vi "test_read-nmea-data2.vi"() -> ()   [LabVIEW 2019] (continued)
\n15:13:53.49\tF9P\t$GLGSV,2,1,08,69,11,031,33,70,70,038,25,71,53,206,32,72,05,210,17,1*72\n\t\n15:13:53.51\tF9P\t$GLGSV,2,2,08,77,01,325,,84,19,123,24,85,70,070,34,86,37,330,,1*77\n\t\n15:13:53.53\tF9P\t$GLGSV,2,1,08,69,11,031,31,70,70,038,,71,53,206,25,72,05,210,,3*75\n\t\n15:13:53.55\tF9P\t$GLGSV,2,2,08,77,01,325,,84,19,123,30,85,70,070,24,86,37,330,,3*71\n\t\n15:13:53.57\tF9P\t$GAGSV,2,1,08,02,08,296,12,04,67,115,32,09,32,193,20,11,72,359,26,7*72\n\t\n15:13:53.59\tF9P\t$GAGSV,2,2,08,12,40,103,28,19,26,045,19,25,09,249,10,36,26,308,12,7*78\n\t\n15:13:53.61\tF9P\t$GAGSV,2,1,08,02,08,296,,04,67,115,,09,32,193,,11,72,359,,2*73\n\t\n15:13:53.63\tF9P\t$GAGSV,2,2,08,12,40,103,,19,26,045,,25,09,249,,36,26,308,,2*7D\n\t\n15:13:53.65\tF9P\t$GBGSV,1,1,04,11,49,132,36,14,87,114,26,28,,,27,33,61,220,30,1*4B\n\t\n15:13:53.67\tF9P\t$GBGSV,1,1,03,11,49,132,33,14,87,114,,33,61,220,,3*43\n\t\n15:13:53.69\tF9P\t$GNGLL,3723.57673,N,12656.98677,E,061355.00,A,A*77\n\t\n15:13:53.71\tF9P\t\t\n15:13:53.73\tF9P\t\t\n15:13:53.75\tF9P\t\t\n15:13:53.77\tF9P\t\t\n15:13:53.79\tF9P\t\t\n15:13:53.81\tF9P\t\t\n15:13:53.83\tF9P\t\t\n15:13:53.85\tF9P\t\t\n15:13:53.87\tF9P\t\t\n15:13:53.89\tF9P\t\t\n15:13:53.91\tF9P\t\t\n15:13:53.93\tF9P\t\t\n15:13:53.95\tF9P\t\t\n15:13:53.97\tF9P\t\t\n15:13:53.99\tF9P\t\t\n15:13:54.01\tF9P\t\t\n15:13:54.03\tF9P\t\t\n15:13:54.05\tF9P\t\t\n15:13:54.07\tF9P\t\t\n15:13:54.09\tF9P\t\t\n15:13:54.11\tF9P\t\t\n15:13:54.13\tF9P\t\t\n15:13:54.15\tF9P\t\t\n15:13:54.17\tF9P\t\t\n15:13:54.19\tF9P\t\t\n15:13:54.21\tF9P\t\t\n15:13:54.23\tF9P\t$GNRMC,061356.00,A,3723.57755,N,12656.98651,E,2.289,328.38,250720,,,A,V*09\n\t\n15:13:54.25\tF9P\t$GNVTG,328.38,T,,M,2.289,N,4.239,K,A*2C\n\t\n15:13:54.27\tF9P\t$GNGGA,061356.00,3723.57755,N,12656.98651,E,1,12,0.74,48.4,M,18.5,M,,*74\n\t\n15:13:54.29\tF9P\t$GNGSA,A,3,12,06,19,05,17,09,04,02,,,,,1.37,0.74,1.15,1*03\n\t\n15:13:54.31\tF9P\t$GNGSA,A,3,85,70,71,84,,,,,,,,,1.37,0.74,1.15,2*01\n\t\n15:13:54.33\tF9P\t$GNGSA,A,3,36,19,11,04,09,12,,,,,,,1.37,0.74,1.15,3*03\n\t\n15:13:54.35\tF9P\t$GNGSA,A,3,14,11,33,,,,,,,,,,1.37,0.74,1.15,4*02\n\t\n15:13:54.37\tF9P\t$GPGSV,3,1,09,02,55,320,27,04,17,043,23,05,38,248,23,06,64,050,29,1*66\n\t\n15:13:54.39\tF9P\t$GPGSV,3,2,09,09,44,073,29,12,23,276,25,17,32,154,33,19,51,157,35,1*62\n\t\n15:13:54.41\tF9P\t$GPGSV,3,3,09,25,12,306,23,1*5D\n\t\n15:13:54.43\tF9P\t$GPGSV,3,1,09,02,55,320,,04,17,043,,05,38,248,18,06,64,050,23,6*67\n\t\n15:13:54.45\tF9P\t$GPGSV,3,2,09,09,44,073,30,12,23,276,,17,32,154,19,19,51,157,,6*64\n\t\n15:13:54.47\tF9P\t$GPGSV,3,3,09,25,12,306,,6*5B\n\t\n15:13:54.49\tF9P\t$GLGSV,2,1,08,69,11,031,34,70,70,038,25,71,53,206,32,72,05,210,17,1*75\n\t\n15:13:54.51\tF9P\t$GLGSV,2,2,08,77,01,325,,84,19,123,26,85,70,070,39,86,37,330,,1*78\n\t\n15:13:54.53\tF9P\t$GLGSV,2,1,08,69,11,031,26,70,70,038,,71,53,206,23,72,05,210,,3*75\n\t\n15:13:54.55\tF9P\t$GLGSV,2,2,08,77,01,325,,84,19,123,33,85,70,070,23,86,37,330,,3*75\n\t\n15:13:54.57\tF9P\t$GAGSV,2,1,08,02,08,296,10,04,67,115,40,09,32,193,21,11,72,359,26,7*74\n\t\n15:13:54.59\tF9P\t$GAGSV,2,2,08,12,40,103,33,19,26,045,20,25,09,249,13,36,26,308,13,7*7A\n\t\n15:13:54.61\tF9P\t$GAGSV,2,1,08,02,08,296,,04,67,115,,09,32,193,,11,72,359,,2*73\n\t\n15:13:54.63\tF9P\t$GAGSV,2,2,08,12,40,103,,19,26,045,,25,09,249,,36,26,308,,2*7D\n\t\n15:13:54.65\tF9P\t$GBGSV,1,1,04,11,49,132,30,14,87,114,32,28,,,25,33,61,220,29,1*42\n\t\n15:13:54.67\tF9P\t$GBGSV,1,1,03,11,49,132,32,14,87,114,29,33,61,220,,3*49\n\t\n15:13:54.69\tF9P\t$GNGLL,3723.57755,N,12656.98651,E,061356.00,A,A*75\n\t\n15:13:54.71\tF9P\t\t\n15:13:54.73\tF9P\t\t\n15:13:54.75\tF9P\t\t\n15:13:54.77\tF9P\t\t\n15:13:54.79\tF9P\t\t\n15:13:54.81\tF9P\t\t\n15:13:54.83\tF9P\t\t\n15:13:54.85\tF9P\t\t\n15:13:54.87\tF9P\t\t\n15:13:54.89\tF9P\t\t\n15:13:54.91\tF9P\t\t\n15:13:54.93\tF9P\t\t\n15:13:54.95\tF9P\t\t\n15:13:54.97\tF9P\t\t\n15:13:54.99\tF9P\t\t\n15:13:55.01\tF9P\t\t\n15:13:55.03\tF9P\t\t\n15:13:55.05\tF9P\t\t\n15:13:55.07\tF9P\t\t\n15:13:55.09\tF9P\t\t\n15:13:55.11\tF9P\t\t\n15:13:55.13\tF9P\t\t\n15:13:55.15\tF9P\t\t\n15:13:55.17\tF9P\t\t\n15:13:55.19\tF9P\t\t\n15:13:55.21\tF9P\t\t\n15:13:55.23\tF9P\t$GNRMC,061357.00,A,3723.57810,N,12656.98637,E,2.065,333.34,250720,,,A,V*00\n\t\n15:13:55.25\tF9P\t$GNVTG,333.34,T,,M,2.065,N,3.825,K,A*2A\n\t\n15:13:55.27\tF9P\t$GNGGA,061357.00,3723.57810,N,12656.98637,E,1,12,0.70,48.3,M,18.5,M,,*78\n\t\n15:13:55.29\tF9P\t$GNGSA,A,3,12,06,19,05,17,09,04,02,,,,,1.27,0.70,1.06,1*04\n\t\n15:13:55.31\tF9P\t$GNGSA,A,3,85,70,71,84,,,,,,,,,1.27,0.70,1.06,2*06\n\t\n15:13:55.33\tF9P\t$GNGSA,A,3,36,19,11,04,09,12,,,,,,,1.27,0.70,1.06,3*04\n\t\n15:13:55.35\tF9P\t$GNGSA,A,3,14,11,33,,,,,,,,,,1.27,0.70,1.06,4*05\n\t\n15:13:55.37\tF9P\t$GPGSV,3,1,09,02,55,320,25,04,17,043,24,05,38,248,34,06,64,050,29,1*65\n\t\n15:13:55.39\tF9P\t$GPGSV,3,2,09,09,44,073,29,12,23,276,25,17,32,154,40,19,51,157,28,1*6A\n\t\n15:13:55.41\tF9P\t$GPGSV,3,3,09,25,12,306,19,1*54\n\t\n15:13:55.43\tF9P\t$GPGSV,3,1,09,02,55,320,,04,17,043,20,05,38,248,20,06,64,050,22,6*6F\n\t\n15:13:55.45\tF9P\t$GPGSV,3,2,09,09,44,073,23,12,23,276,,17,32,154,23,19,51,157,,6*6F\n\t\n15:13:55.47\tF9P\t$GPGSV,3,3,09,25,12,306,,6*5B\n\t\n15:13:55.49\tF9P\t$GLGSV,2,1,08,69,11,031,26,70,70,038,24,71,53,206,27,72,05,210,17,1*73\n\t\n15:13:55.51\tF9P\t$GLGSV,2,2,08,77,01,325,,84,19,123,31,85,70,070,32,86,37,330,,1*75\n\t\n15:13:55.53\tF9P\t$GLGSV,2,1,08,69,11,031,25,70,70,038,,71,53,206,22,72,05,210,,3*77\n\t\n15:13:55.55\tF9P\t$GLGSV,2,2,08,77,01,325,,84,19,123,32,85,70,070,22,86,37,330,,3*75\n\t\n15:13:55.57\tF9P\t$GAGSV,2,1,08,02,08,296,10,04,67,115,27,09,33,193,21,11,72,359,26,7*74\n\t\n15:13:55.59\tF9P\t$GAGSV,2,2,08,12,40,103,29,19,26,045,19,25,09,249,15,36,26,308,11,7*7F\n\t\n15:13:55.61\tF9P\t$GAGSV,2,1,08,02,08,296,,04,67,115,,09,33,193,,11,72,359,,2*72\n\t\n15:13:55.63\tF9P\t$GAGSV,2,2,08,12,40,103,,19,26,045,,25,09,249,,36,26,308,,2*7D\n\t\n15:13:55.65\tF9P\t$GBGSV,1,1,04,11,49,132,27,14,87,114,31,28,,,27,33,61,220,36,1*4B\n\t\n15:13:55.67\tF9P\t$GBGSV,1,1,04,08,,,36,11,49,132,32,14,87,114,34,33,61,220,,3*4F\n\t\n15:13:55.69\tF9P\t$GNGLL,3723.57810,N,12656.98637,E,061357.00,A,A*7A\n\t\n15:13:55.71\tF9P\t\t\n15:13:55.73\tF9P\t\t\n15:13:55.75\tF9P\t\t\n15:13:55.77\tF9P\t\t\n15:13:55.79\tF9P\t\t\n15:13:55.81\tF9P\t\t\n15:13:55.83\tF9P\t\t\n15:13:55.85\tF9P\t\t\n15:13:55.87\tF9P\t\t\n15:13:55.89\tF9P\t\t\n15:13:55.91\tF9P\t\t\n15:13:55.93\tF9P\t\t\n15:13:55.95\tF9P\t\t\n15:13:55.97\tF9P\t\t\n15:13:55.99\tF9P\t\t\n15:13:56.01\tF9P\t\t\n15:13:56.03\tF9P\t\t\n15:13:56.05\tF9P\t\t\n15:13:56.07\tF9P\t\t\n15:13:56.09\tF9P\t\t\n15:13:56.11\tF9P\t\t\n15:13:56.13\tF9P\t\t\n15:13:56.15\tF9P\t\t\n15:13:56.17\tF9P\t\t\n15:13:56.19\tF9P\t\t\n15:13:56.21\tF9P\t\t\n15:13:56.23\tF9P\t$GNRMC,061358.00,A,3723.57882,N,12656.98586,E,2.274,334.11,250720,,,A,V*0F\n\t\n15:13:56.25\tF9P\t$GNVTG,334.11,T,,M,2.274,N,4.211,K,A*22\n\t\n15:13:56.27\tF9P\t$GNGGA,061358.00,3723.57882,N,12656.98586,E,1,12,0.74,47.8,M,18.5,M,,*75\n\t\n15:13:56.29\tF9P\t$GNGSA,A,3,12,06,19,05,17,09,04,02,,,,,1.37,0.74,1.15,1*03\n\t\n15:13:56.31\tF9P\t$GNGSA,A,3,85,70,71,84,,,,,,,,,1.37,0.74,1.15,2*01\n\t\n15:13:56.33\tF9P\t$GNGSA,A,3,36,19,11,04,09,12,,,,,,,1.37,0.74,1.15,3*03\n\t\n15:13:56.35\tF9P\t$GNGSA,A,3,14,11,33,,,,,,,,,,1.37,0.74,1.15,4*02\n\t\n15:13:56.37\tF9P\t$GPGSV,3,1,09,02,55,320,25,04,17,043,24,05,38,248,42,06,64,050,33,1*6F\n\t\n15:13:56.39\tF9P\t$GPGSV,3,2,09,09,44,073,33,12,23,276,30,17,32,154,36,19,51,157,33,1*6E\n\t\n15:13:56.41\tF9P\t$GPGSV,3,3,09,25,12,306,18,1*55\n\t\n15:13:56.43\tF9P\t$GPGSV,3,1,09,02,55,320,,04,17,043,18,05,38,248,22,06,64,050,24,6*60\n\t\n15:13:56.45\tF9P\t$GPGSV,3,2,09,09,44,073,23,12,23,276,,17,32,154,22,19,51,157,19,6*66\n\t\n15:13:56.47\tF9P\t$GPGSV,3,3,09,25,12,306,,6*5B\n\t\n15:13:56.49\tF9P\t$GLGSV,2,1,08,69,11,031,30,70,70,038,22,71,53,206,30,72,05,210,17,1*74\n\t\n15:13:56.51\tF9P\t$GLGSV,2,2,08,77,01,325,,84,19,123,28,85,70,070,27,86,37,330,,1*79\n\t\n15:13:56.53\tF9P\t$GLGSV,2,1,08,69,11,031,23,70,70,038,,71,53,206,27,72,05,210,,3*74\n\t\n15:13:56.55\tF9P\t$GLGSV,2,2,08,77,01,325,,84,19,123,35,85,70,070,21,86,37,330,,3*71\n\t\n15:13:56.57\tF9P\t$GAGSV,2,1,08,02,08,296,08,04,67,115,30,09,33,193,22,11,72,001,26,7*76\n\t\n15:13:56.59\tF9P\t$GAGSV,2,2,08,12,40,103,23,19,26,045,21,25,09,249,15,36,26,308,13,7*7C\n\t\n15:13:56.61\tF9P\t$GAGSV,2,1,08,02,08,296,,04,67,115,,09,33,193,,11,72,001,,2*7C\n\t\n15:13:56.63\tF9P\t$GAGSV,2,2,08,12,40,103,,19,26,045,,25,09,249,,36,26,308,,2*7D\n\t\n15:13:56.65\tF9P\t$GBGSV,1,1,04,11,49,132,32,14,87,114,32,28,,,31,33,61,220,36,1*4B\n\t\n15:13:56.67\tF9P\t$GBGSV,1,1,04,08,,,33,11,49,132,30,14,87,114,34,33,61,220,,3*48\n\t\n15:13:56.69\tF9P\t$GNGLL,3723.57882,N,12656.98586,E,061358.00,A,A*77\n\t\n15:13:56.71\tF9P\t\t\n15:13:56.73\tF9P\t\t\n15:13:56.75\tF9P\t\t\n15:13:56.77\tF9P\t\t\n15:13:56.79\tF9P\t\t\n15:13:56.81\tF9P\t\t\n15:13:56.83\tF9P\t\t\n15:13:56.85\tF9P\t\t\n15:13:56.87\tF9P\t\t\n15:13:56.89\tF9P\t\t\n15:13:56.91\tF9P\t\t\n15:13:56.93\tF9P\t\t\n15:13:56.95\tF9P\t\t\n15:13:56.97\tF9P\t\t\n15:13:56.99\tF9P\t\t\n15:13:57.01\tF9P\t\t\n15:13:57.03\tF9P\t\t\n15:13:57.05\tF9P\t\t\n15:13:57.07\tF9P\t\t\n15:13:57.09\tF9P\t\t\n15:13:57.11\tF9P\t\t\n15:13:57.13\tF9P\t\t\n15:13:57.15\tF9P\t\t\n15:13:57.17\tF9P\t\t\n15:13:57.19\tF9P\t\t\n15:13:57.21\tF9P\t\t\n15:13:57.23\tF9P\t$GNRMC,061359.00,A,3723.57946,N,12656.98547,E,2.498,332.08,250720,,,A,V*00\n\t\n15:13:57.25\tF9P\t$GNVTG,332.08,T,,M,2.498,N,4.627,K,A*29\n\t\n15:13:57.27\tF9P\t$GNGGA,061359.00,3723.57946,N,12656.98547,E,1,12,0.74,47.9,M,18.5,M,,*71\n\t\n15:13:57.29\tF9P\t$GNGSA,A,3,12,06,19,05,17,09,04,02,,,,,1.37,0.74,1.15,1*03\n\t\n15:13:57.31\tF9P\t$GNGSA,A,3,85,70,71,84,,,,,,,,,1.37,0.74,1.15,2*01\n\t\n15:13:57.33\tF9P\t$GNGSA,A,3,36,19,11,04,09,12,,,,,,,1.37,0.74,1.15,3*03\n\t\n15:13:57.35\tF9P\t$GNGSA,A,3,14,11,33,,,,,,,,,,1.37,0.74,1.15,4*02\n\t\n15:13:57.37\tF9P\t$GPGSV,3,1,09,02,55,320,28,04,17,043,25,05,38,248,28,06,64,050,40,1*6B\n\t\n15:13:57.39\tF9P\t$GPGSV,3,2,09,09,44,073,29,12,23,276,22,17,32,154,40,19,51,157,22,1*67\n\t\n15:13:57.41\tF9P\t$GPGSV,3,3,09,25,12,306,18,1*55\n\t\n15:13:57.43\tF9P\t$GPGSV,3,1,09,02,55,320,,04,17,043,15,05,38,248,20,06,64,050,22,6*69\n\t\n15:13:57.45\tF9P\t$GPGSV,3,2,09,09,44,073,21,12,23,276,18,17,32,154,21,19,51,157,16,6*61\n\t\n15:13:57.47\tF9P\t$GPGSV,3,3,09,25,12,306,,6*5B\n\t\n15:13:57.49\tF9P\t$GLGSV,2,1,08,69,11,031,28,70,70,038,22,71,53,206,30,72,05,210,18,1*72\n\t\n15:13:57.51\tF9P\t$GLGSV,2,2,08,77,01,325,,84,19,123,29,85,70,070,28,86,37,330,,1*77\n\t\n15:13:57.53\tF9P\t$GLGSV,2,1,08,69,11,031,22,70,70,038,,71,53,206,25,72,05,210,,3*77\n\t\n15:13:57.55\tF9P\t$GLGSV,2,2,08,77,01,325,,84,19,123,25,85,70,070,21,86,37,330,,3*70\n\t\n15:13:57.57\tF9P\t$GAGSV,2,1,08,02,08,296,09,04,67,115,23,09,33,193,22,11,72,001,26,7*75\n\t\n15:13:57.59\tF9P\t$GAGSV,2,2,08,12,39,103,25,19,26,045,21,25,09,249,16,36,26,308,12,7*76\n\t\n15:13:57.61\tF9P\t$GAGSV,2,1,08,02,08,296,,04,67,115,,09,33,193,,11,72,001,,2*7C\n\t\n15:13:57.63\tF9P\t$GAGSV,2,2,08,12,39,103,,19,26,045,,25,09,249,,36,26,308,,2*73\n\t\n15:13:57.65\tF9P\t$GBGSV,1,1,04,11,49,132,35,14,87,114,28,28,,,25,33,61,220,32,1*46\n\t\n15:13:57.67\tF9P\t$GBGSV,1,1,04,08,,,30,11,49,132,26,14,87,114,31,33,61,220,,3*49\n\t\n15:13:57.69\tF9P\t$GNGLL,3723.57946,N,12656.98547,E,061359.00,A,A*72\n\t\n15:13:57.71\tF9P\t\t\n15:13:57.73\tF9P\t\t\n15:13:57.75\tF9P\t\t\n15:13:57.77\tF9P\t\t\n15:13:57.79\tF9P\t\t\n15:13:57.81\tF9P\t\t\n15:13:57.83\tF9P\t\t\n15:13:57.85\tF9P\t\t\n15:13:57.87\tF9P\t\t\n15:13:57.89\tF9P\t\t\n15:13:57.91\tF9P\t\t\n15:13:57.93\tF9P\t\t\n15:13:57.95\tF9P\t\t\n15:13:57.97\tF9P\t\t\n15:13:57.99\tF9P\t\t\n15:13:58.01\tF9P\t\t\n15:13:58.03\tF9P\t\t\n15:13:58.05\tF9P\t\t\n15:13:58.07\tF9P\t\t\n15:13:58.09\tF9P\t\t\n15:13:58.11\tF9P\t\t\n15:13:58.13\tF9P\t\t\n15:13:58.15\tF9P\t\t\n15:13:58.17\tF9P\t\t\n15:13:58.19\tF9P\t\t\n15:13:58.21\tF9P\t\t\n15:13:58.23\tF9P\t$GNRMC,061400.00,A,3723.58004,N,12656.98518,E,1.633,332.76,250720,,,A,V*08\n\t\n15:13:58.25\tF9P\t$GNVTG,332.76,T,,M,1.633,N,3.024,K,A*22\n\t\n15:13:58.27\tF9P\t$GNGGA,061400.00,3723.58004,N,12656.98518,E,1,12,0.71,47.9,M,18.5,M,,*75\n\t\n15:13:58.29\tF9P\t$GNGSA,A,3,12,06,19,05,17,09,04,02,,,,,1.33,0.71,1.12,1*05\n\t\n15:13:58.31\tF9P\t$GNGSA,A,3,85,70,71,84,,,,,,,,,1.33,0.71,1.12,2*07\n\t\n15:13:58.33\tF9P\t$GNGSA,A,3,36,19,11,04,09,12,,,,,,,1.33,0.71,1.12,3*05\n\t\n15:13:58.35\tF9P\t$GNGSA,A,3,14,11,33,,,,,,,,,,1.33,0.71,1.12,4*04\n\t\n15:13:58.37\tF9P\t$GPGSV,3,1,09,02,55,320,28,04,17,043,25,05,38,248,41,06,64,050,29,1*6B\n\t\n15:13:58.39\tF9P\t$GPGSV,3,2,09,09,44,073,32,12,23,276,21,17,32,154,30,19,51,157,28,1*63\n\t\n15:13:58.41\tF9P\t$GPGSV,3,3,09,25,12,306,19,1*54\n\t\n15:13:58.43\tF9P\t$GPGSV,3,1,09,02,55,320,,04,17,043,16,05,38,248,29,06,64,050,30,6*60\n\t\n15:13:58.45\tF9P\t$GPGSV,3,2,09,09,44,073,20,12,23,276,15,17,32,154,21,19,51,157,09,6*63\n\t\n15:13:58.47\tF9P\t$GPGSV,3,3,09,25,12,306,,6*5B\n\t\n15:13:58.49\tF9P\t$GLGSV,2,1,08,69,11,031,22,70,70,038,22,71,53,206,23,72,05,210,17,1*75\n\t\n15:13:58.51\tF9P\t$GLGSV,2,2,08,77,01,325,,84,19,123,27,85,70,070,32,86,37,330,,1*72\n\t\n15:13:58.53\tF9P\t$GLGSV,2,1,08,69,11,031,25,70,70,038,,71,53,206,23,72,05,210,,3*76\n\t\n15:13:58.55\tF9P\t$GLGSV,2,2,08,77,01,325,,84,19,123,26,85,70,070,21,86,37,330,,3*73\n\t\n15:13:58.57\tF9P\t$GAGSV,2,1,08,02,08,296,10,04,67,115,25,09,33,193,30,11,72,001,26,7*78\n\t\n15:13:58.59\tF9P\t$GAGSV,2,2,08,12,39,103,24,19,26,045,21,25,09,249,14,36,26,308,14,7*73\n\t\n15:13:58.61\tF9P\t$GAGSV,2,1,08,02,08,296,,04,67,115,,09,33,193,,11,72,001,31,2*7E\n\t\n15:13:58.63\tF9P\t$GAGSV,2,2,08,12,39,103,,19,26,045,,25,09,249,,36,26,308,,2*73\n\t\n15:13:58.65\tF9P\t$GBGSV,1,1,04,11,49,132,28,14,87,114,26,28,,,25,33,61,220,37,1*41\n\t\n15:13:58.67\tF9P\t$GBGSV,1,1,04,08,,,29,11,49,132,,14,87,114,30,33,61,220,,3*44\n\t\n15:13:58.70\tF9P\t$GNGLL,3723.58004,N,12656.98518,E,061400.00,A,A*73\n\t\n15:13:58.72\tF9P\t\t\n15:13:58.74\tF9P\t\t\n15:13:58.76\tF9P\t\t\n15:13:58.78\tF9P\t\t\n15:13:58.80\tF9P\t\t\n15:13:58.82\tF9P\t\t\n15:13:58.84\tF9P\t\t\n15:13:58.86\tF9P\t\t\n15:13:58.88\tF9P\t\t\n15:13:58.90\tF9P\t\t\n15:13:58.92\tF9P\t\t\n15:13:58.94\tF9P\t\t\n15:13:58.96\tF9P\t\t\n15:13:58.98\tF9P\t\t\n15:13:59.00\tF9P\t\t\n15:13:59.02\tF9P\t\t\n15:13:59.04\tF9P\t\t\n15:13:59.06\tF9P\t\t\n15:13:59.08\tF9P\t\t\n15:13:59.10\tF9P\t\t\n15:13:59.12\tF9P\t\t\n15:13:59.14\tF9P\t\t\n15:13:59.16\tF9P\t\t\n15:13:59.18\tF9P\t\t\n15:13:59.20\tF9P\t\t\n15:13:59.22\tF9P\t\t\n15:13:59.24\tF9P\t$GNRMC,061401.00,A,3723.58046,N,12656.98492,E,0.886,335.81,250720,,,A,V*02\n\t\n15:13:59.26\tF9P\t$GNVTG,335.81,T,,M,0.886,N,1.641,K,A*2B\n\t\n15:13:59.28\tF9P\t$GNGGA,061401.00,3723.58046,N,12656.98492,E,1,12,0.71,47.5,M,18.5,M,,*7D\n\t\n15:13:59.30\tF9P\t$GNGSA,A,3,12,06,19,05,17,09,04,02,,,,,1.27,0.71,1.05,1*06\n\t\n15:13:59.32\tF9P\t$GNGSA,A,3,85,70,71,84,,,,,,,,,1.27,0.71,1.05,2*04\n\t\n15:13:59.34\tF9P\t$GNGSA,A,3,36,19,11,04,09,12,,,,,,,1.27,0.71,1.05,3*06\n\t\n15:13:59.36\tF9P\t$GNGSA,A,3,14,11,33,,,,,,,,,,1.27,0.71,1.05,4*07\n\t\n15:13:59.38\tF9P\t$GPGSV,3,1,09,02,55,320,32,04,17,043,26,05,38,248,42,06,64,050,28,1*61\n\t\n15:13:59.40\tF9P\t$GPGSV,3,2,09,09,44,073,33,12,23,276,22,17,32,154,30,19,51,157,27,1*6E\n\t\n15:13:59.42\tF9P\t$GPGSV,3,3,09,25,12,306,18,1*55\n\t\n15:13:59.44\tF9P\t$GPGSV,3,1,09,02,55,320,,04,17,043,19,05,38,248,20,06,64,050,22,6*65\n\t\n15:13:59.46\tF9P\t$GPGSV,3,2,09,09,44,073,23,12,23,276,12,17,32,154,21,19,51,157,08,6*66\n\t\n15:13:59.48\tF9P\t$GPGSV,3,3,09,25,12,306,,6*5B\n\t\n15:13:59.50\tF9P\t$GLGSV,2,1,08,69,11,031,24,70,70,038,24,71,53,206,31,72,05,210,15,1*74\n\t\n15:13:59.52\tF9P\t$GLGSV,2,2,08,77,01,325,,84,19,123,10,85,70,070,33,86,37,330,,1*77\n\t\n15:13:59.54\tF9P\t$GLGSV,2,1,08,69,11,031,23,70,70,038,,71,53,206,26,72,05,210,,3*75\n\t\n15:13:59.56\tF9P\t$GLGSV,2,2,08,77,01,325,,84,19,123,25,85,70,070,20,86,37,330,,3*71\n\t\n15:13:59.58\tF9P\t$GAGSV,2,1,08,02,08,296,11,04,67,115,31,09,33,193,23,11,72,001,34,7*7D\n\t\n15:13:59.60\tF9P\t$GAGSV,2,2,08,12,39,103,24,19,26,045,23,25,09,249,11,36,26,308,17,7*77\n\t\n15:13:59.62\tF9P\t$GAGSV,2,1,08,02,08,296,,04,67,115,,09,33,193,,11,72,001,,2*7C\n\t\n15:13:59.64\tF9P\t$GAGSV,2,2,08,12,39,103,,19,26,045,,25,09,249,,36,26,308,,2*73\n\t\n15:13:59.66\tF9P\t$GBGSV,1,1,04,11,49,132,28,14,87,114,32,28,,,31,33,61,220,26,1*41\n\t\n15:13:59.68\tF9P\t$GBGSV,1,1,04,08,,,33,11,49,132,26,14,87,114,29,33,61,220,,3*43\n\t\n15:13:59.70\tF9P\t$GNGLL,3723.58046,N,12656.98492,E,061401.00,A,A*77\n\t\n15:13:59.72\tF9P\t\t\n15:13:59.74\tF9P\t\t\n15:13:59.76\tF9P\t\t\n15:13:59.78\tF9P\t\t\n15:13:59.80\tF9P\t\t\n15:13:59.82\tF9P\t\t\n15:13:59.84\tF9P\t\t\n15:13:59.86\tF9P\t\t\n15:13:59.88\tF9P\t\t\n15:13:59.90\tF9P\t\t\n15:13:59.92\tF9P\t\t\n15:13:59.94\tF9P\t\t\n15:13:59.96\tF9P\t\t\n15:13:59.98\tF9P\t\t\n15:14:00.00\tF9P\t\t\n15:14:00.02\tF9P\t\t\n15:14:00.04\tF9P\t\t\n15:14:00.06\tF9P\t\t\n15:14:00.08\tF9P\t\t\n15:14:00.10\tF9P\t\t\n15:14:00.12\tF9P\t\t\n15:14:00.14\tF9P\t\t\n15:14:00.16\tF9P\t\t\n15:14:00.18\tF9P\t\t\n15:14:00.20\tF9P\t\t\n15:14:00.22\tF9P\t\t\n15:14:00.24\tF9P\t$GNRMC,061402.00,A,3723.58095,N,12656.98450,E,1.833,322.52,250720,,,A,V*06\n\t\n15:14:00.26\tF9P\t$GNVTG,322.52,T,,M,1.833,N,3.394,K,A*23\n\t\n15:14:00.28\tF9P\t$GNGGA,061402.00,3723.58095,N,12656.98450,E,1,12,0.71,47.8,M,18.5,M,,*73\n\t\n15:14:00.30\tF9P\t$GNGSA,A,3,12,06,19,05,17,09,04,02,,,,,1.27,0.71,1.05,1*06\n\t\n15:14:00.32\tF9P\t$GNGSA,A,3,85,70,71,84,,,,,,,,,1.27,0.71,1.05,2*04\n\t\n15:14:00.34\tF9P\t$GNGSA,A,3,36,19,11,04,09,12,,,,,,,1.27,0.71,1.05,3*06\n\t\n15:14:00.36\tF9P\t$GNGSA,A,3,14,11,33,,,,,,,,,,1.27,0.71,1.05,4*07\n\t\n15:14:00.38\tF9P\t$GPGSV,3,1,09,02,55,320,28,04,17,043,25,05,38,248,25,06,64,050,27,1*67\n\t\n15:14:00.40\tF9P\t$GPGSV,3,2,09,09,44,073,32,12,23,276,22,17,32,154,36,19,51,157,28,1*66\n\t\n15:14:00.42\tF9P\t$GPGSV,3,3,09,25,12,306,16,1*5B\n\t\n15:14:00.44\tF9P\t$GPGSV,3,1,09,02,55,320,,04,17,043,19,05,38,248,18,06,64,050,23,6*6F\n\t\n15:14:00.46\tF9P\t$GPGSV,3,2,09,09,44,073,22,12,23,276,12,17,32,154,19,19,51,157,,6*64\n\t\n15:14:00.48\tF9P\t$GPGSV,3,3,09,25,12,306,,6*5B\n\t\n15:14:00.50\tF9P\t$GLGSV,2,1,08,69,11,031,24,70,70,038,26,71,53,206,25,72,05,210,,1*77\n\t\n15:14:00.52\tF9P\t$GLGSV,2,2,08,77,01,325,,84,19,123,16,85,70,070,30,86,37,330,,1*72\n\t\n15:14:00.54\tF9P\t$GLGSV,2,1,08,69,11,031,19,70,70,038,,71,53,206,22,72,05,210,,3*78\n\t\n15:14:00.56\tF9P\t$GLGSV,2,2,08,77,01,325,,84,19,123,23,85,70,070,22,86,37,330,,3*75\n\t\n15:14:00.58\tF9P\t$GAGSV,2,1,08,02,08,296,10,04,67,115,30,09,33,193,22,11,72,001,30,7*78\n\t\n15:14:00.60\tF9P\t$GAGSV,2,2,08,12,39,103,22,19,25,045,23,25,09,249,,36,26,308,11,7*74\n\t\n15:14:00.62\tF9P\t$GAGSV,2,1,08,02,08,296,,04,67,115,26,09,33,193,,11,72,001,,2*78\n\t\n15:14:00.64\tF9P\t$GAGSV,2,2,08,12,39,103,,19,25,045,,25,09,249,,36,26,308,,2*70\n\t\n15:14:00.66\tF9P\t$GBGSV,1,1,04,11,49,132,28,14,87,114,27,28,,,24,33,61,220,27,1*40\n\t\n15:14:00.68\tF9P\t$GBGSV,1,1,04,08,,,29,11,49,132,27,14,87,114,27,33,61,220,,3*47\n\t\n15:14:00.70\tF9P\t$GNGLL,3723.58095,N,12656.98450,E,061402.00,A,A*74\n\t\n15:14:00.72\tF9P\t\t\n15:14:00.74\tF9P\t\t\n15:14:00.76\tF9P\t\t\n15:14:00.78\tF9P\t\t\n15:14:00.80\tF9P\t\t\n15:14:00.82\tF9P\t\t\n15:14:00.84\tF9P\t\t\n15:14:00.86\tF9P\t\t\n15:14:00.88\tF9P\t\t\n15:14:00.90\tF9P\t\t\n15:14:00.92\tF9P\t\t\n15:14:00.94\tF9P\t\t\n15:14:00.96\tF9P\t\t\n15:14:00.98\tF9P\t\t\n15:14:01.00\tF9P\t\t\n15:14:01.02\tF9P\t\t\n15:14:01.04\tF9P\t\t\n15:14:01.06\tF9P\t\t\n15:14:01.08\tF9P\t\t\n15:14:01.10\tF9P\t\t\n15:14:01.12\tF9P\t\t\n15:14:01.14\tF9P\t\t\n15:14:01.16\tF9P\t\t\n15:14:01.18\tF9P\t\t\n15:14:01.20\tF9P\t\t\n15:14:01.22\tF9P\t\t\n15:14:01.24\tF9P\t$GNRMC,061403.00,A,3723.58118,N,12656.98443,E,0.718,,250720,,,A,V*1C\n\t\n15:14:01.26\tF9P\t$GNVTG,,T,,M,0.718,N,1.329,K,A*3A\n\t\n15:14:01.28\tF9P\t$GNGGA,061403.00,3723.58118,N,12656.98443,E,1,12,0.66,48.0,M,18.5,M,,*75\n\t\n15:14:01.30\tF9P\t$GNGSA,A,3,12,06,19,05,17,09,04,02,,,,,1.18,0.66,0.97,1*06\n\t\n15:14:01.32\tF9P\t$GNGSA,
